vi "GLOBAL_trial_sequence.vi"() -> ()   [LabVIEW 2016]
panel:
  in  "Trial sequence":cluster{"Sequence name":string, "Active":bool}[](array[cluster])
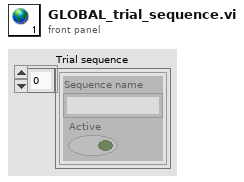
[diagram p1: front panel]
diagram:
